vi "Sequencer.vi"(0 "Test (Default) en entrée":refnum<class "Sequencer (Default).lvclass">, 11 "error in (no error)":errorcluster caption="entrée d'erreur (pas d'erreur)") -> (4 "Test (Default) en sortie":refnum<class "Sequencer (Default).lvclass">, 6 "Json_String":string, 8 "Result":bool, 10 "Result Sequence":T3(array[cluster]), 15 "error out":errorcluster caption="sortie d'erreur")   [LabVIEW 2020, in "Library Core.lvlib" / "Sequencer (Default).lvclass"]
uses:
  Sequencer (Default).lvclass
  Commun VI/TypeDef/Commande Test/Commande Value Type.ctl
  Commun VI/TypeDef/Commande Test/Commande Type Test.ctl
  Actor Test (Default)/Actor Test (Default).lvclass
  Sequencer (Default).lvclass/Sequencer (Default).ctl
  Commun VI/TypeDef/Variable Printable.ctl
  Actor Test Firebase/Actor Test Firebase.lvclass
  C:/Users/ngarcin/OneDrive - Altyor/Standard TB/Suite TB45/Class/Sequencer/Actor Test (Default)/Actor Test (Default).lvclass
  Actor Test Database/Actor Test Database.lvclass
  Variable Test.vi
  Commun VI/Library Commun.lvlib
panel:
  out "Stop in progress":bool
  in  "Default":refnum<class "Actor Test (Default).lvclass">
  out "Numérique":i32
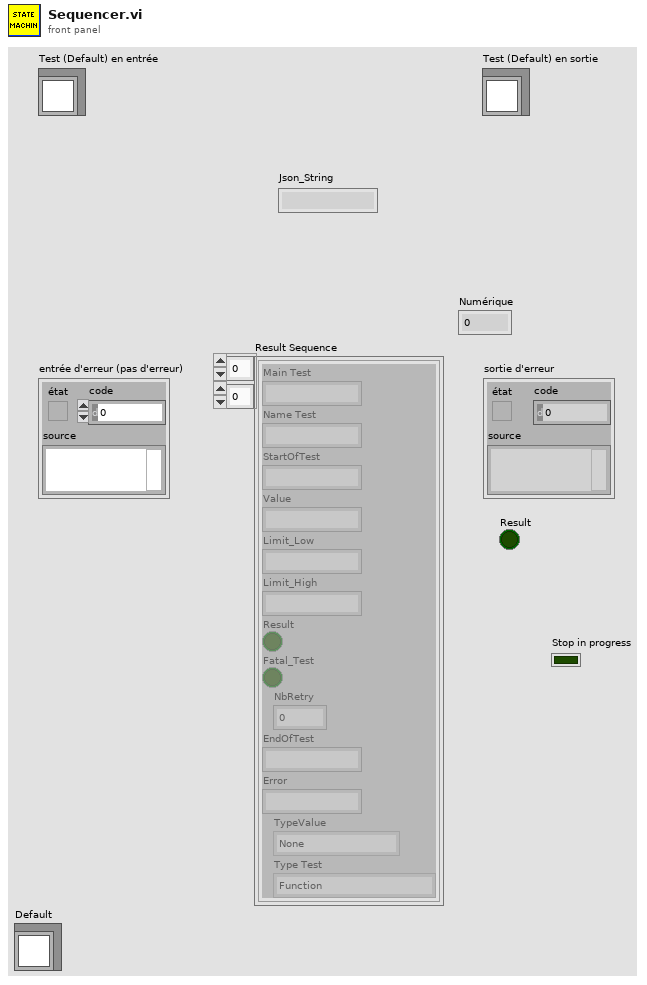
[diagram p1: front panel]
types:
  T1 = typedef "Library Commun.lvlib/Commande Value Type.ctl" = enum16{"None", "String", "Number", "Timestamp", "Boolean", "Array"}
  T2 = typedef "Library Commun.lvlib/Commande Type Test.ctl" = enum16{"Function", "Test", "Calculation"}
  T3 = cluster{"Main Test":string, "Name Test":string, "StartOfTest":string, "Value":string, "Limit_Low":string, "Limit_High":string, "Result":bool, "Fatal_Test":bool, "NbRetry":dbl, "EndOfTest":string, "Error":string, "TypeValue":T1, "Type Test":T2}[][]
  T4 = typedef "Variable Printable.ctl" = string
  T5 = enum16{"Get Variable", "Get All Variables", "Set Variable", "Delete Variable", "Delete All Variable"}
  T6 = enum16{"Get Actor Class", "Set Actor object", "Get Actor object", "List Actor", "Init"}
  T7 = typedef "Library Commun.lvlib/Actor Type.ctl" = enum16{"Default", "Firebase", "Database"}
  T8 = cluster{"Group Name":string, "Tab Test":cluster{"Type Function":string, "Test Name":string, "Class launched by the actors ":string, "Name_Instrument":string, "Class_Instrument":string, "Parameter (Json)":string, "Limit_Low":string, "Limit_Hight":string, "Fatal Test ?":bool, "Parallelized ?":bool, "Mandatory ?":bool}[], "Parallelized ?":bool, "Mandatory ?":bool}[]
  T9 = cluster{"Event Error":refnum<user-event>, "Data test ":refnum<user-event>, "Stop":refnum<user-event>, "Action in progress":refnum<user-event>, "Operator Shutdown":refnum<user-event>}
  T10 = cluster{"Type Function":string, "Test Name":string, "Class launched by the actors ":string, "Name_Instrument":string, "Class_Instrument":string, "Parameter (Json)":string, "Limit_Low":string, "Limit_Hight":string, "Fatal Test ?":bool, "Parallelized ?":bool, "Mandatory ?":bool}[]
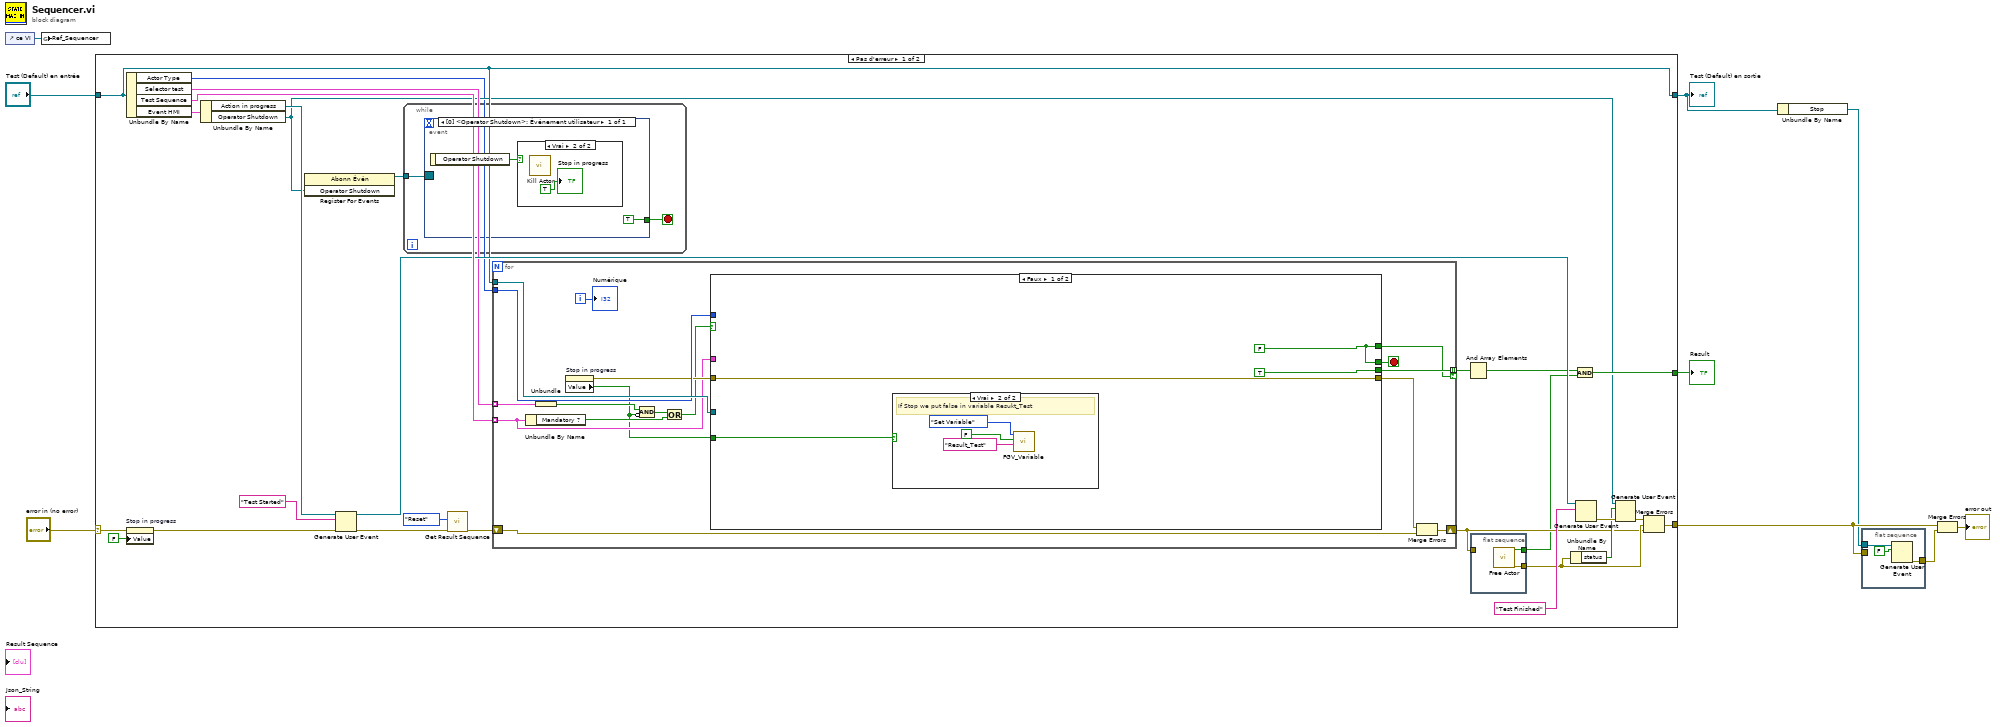
[diagram p0: block diagram]
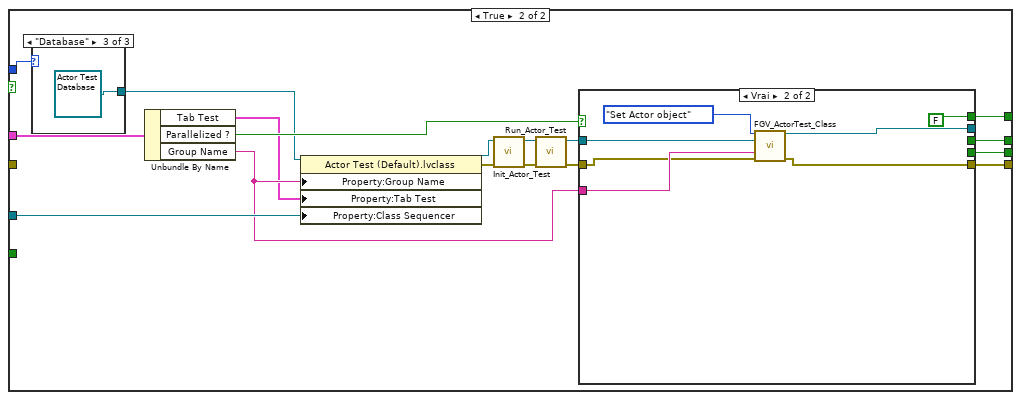
[diagram p3: hidden frame]
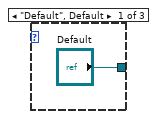
[diagram p4: hidden frame]
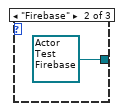
[diagram p5: hidden frame]
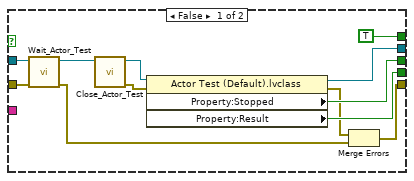
[diagram p6: hidden frame]
diagram:
  n1 = control-ref of="ce VI"() -> (w7:refnum<vi>)
  n2 = global write "Variable Test.vi" "Ref_Sequencer"(w7) -> ()
  n3 = case shown="Pas d'erreur" "error in (no error)" {
    selector: "error in (no error)" -> [w19 w108]
    tunnel: [w22 w108] -> w5
    tunnel: [w30 w107] -> w6
    tunnel: "Test (Default) en entrée" -> [w30 w107]
    tunnel: [w29 _] -> w2
    frame No Error {
      n4 = Unbundle By Name(w30) -> ("Actor Type"=w23:T7, "Selector test"=w28:cluster{"Booléen 4":bool}[], "Test Sequence"=w36:T8, "Event HMI"=w31:T9)
      n5 = property on="Stop in progress" class="Bool (strict)"(error in=w19, "Value"=FALSE ("Stop in progress")) -> (error out=w18:errorcluster)  [unwired: 1 in, 1 out]
      n6 = Unbundle By Name(w31) -> ("Action in progress"=w35:refnum<user-event>, "Operator Shutdown"=w24:refnum<user-event>)
      n7 = register-events(w24) -> (reference out=w27:refnum<event-registration>)  [unwired: 2 in, 1 out]
      n8 = Generate User Event(user event=w35, event data cluster="Test Started" ("données d'événement"), error in=w18) -> (user event out=w33:refnum<user-event>, error out=w15:errorcluster)  [unwired: 1 in]
      n9 = while {
        tunnel: w27 -> [w103]
        stop <- w102 stop-if-true
        n10 = event shown="[0] <Operator Shutdown>: Événement utilisateur" {
          selector: w103 -> [_]
          dyn-events: _ -> [_]
          timeout: _ -> [_]
          tunnel: [TRUE] -> w102
          event User Event {
            n11 = event-data() -> ("Operator Shutdown"=w105:bool)  [unwired: 1 in]
            n12 = case shown="Vrai" w105 {
              frame False {
              }
              frame True {
                n13 = call "Kill Actor.vi"() -> ()  [unwired: 11 in, 1 out]
                "Stop in progress" <- TRUE ("notification")
              }
            }
          }
        }
      }
      n14 = call "Get Result Sequence.vi"("error in (no error)"=w15, "Function"=enum16{"Get Result", "Reset", "Set Result"}."Reset") -> ("error out"=w14:errorcluster)  [unwired: 8 in, 1 out]
      n15 = for {
        shift-right: [w42] -> w13
        shift-left: w14 -> [w41]
        tunnel: w36 -> [w47] mode=indexing
        tunnel: w30 -> [w55]
        tunnel: w28 -> [w54] mode=indexing
        tunnel: [w52] -> w10 mode=indexing if=w51
        tunnel: w23 -> [w49]
        i -> [w50]
        stop <- w53 stop-if-true
        n16 = Unbundle By Name(w47) -> ("Mandatory ?"=w45:bool)
        n17 = Unbundle(w54) -> ("Booléen 4"=w40:bool)
        n18 = property on="Stop in progress" class="Bool (strict)"() -> (error out=w48:errorcluster, "Value"=w39:bool)  [unwired: 2 in, 1 out]
        n19 = Compound Arithmetic op=AND ("Opérateur arithmétique")(w40, invert w39) -> (w46:bool)
        n20 = Or(x=w46, y=w45) -> (x .or. y?=w44:bool)
        n21 = case shown="Faux" w44 {
          tunnel: w47 -> [_ w79]
          tunnel: w48 -> [w59 _]
          tunnel: w55 -> [_ w72]
          tunnel: [w59 w66] -> w43
          tunnel: [w57 w70] -> w53
          tunnel: [TRUE ("Property:Result") w71] -> w52
          tunnel: [w57 w69] -> w51
          tunnel: w49 -> [_ w64]
          tunnel: w39 -> [w56 _]
          frame False {
            w57 = FALSE ("Property:Stopped")
            n22 = case shown="Vrai" w56 {
              frame False {
              }
              frame True {
                # "If Stop we put false in variable Resukt_Test"
                n23 = call "FGV_Variable.vi"("Variable"=T4 "Result_Test", "Data In"=FALSE ("Affiche result"), "Function"=T5."Set Variable") -> ()  [unwired: 6 in, 3 out]
              }
            }
          }
          frame True {
            n24 = case shown="\"Database\"" w64 {
              tunnel: ["Default" refnum<class "Actor Test Firebase.lvclass"> refnum ("Library Sequencer.lvlib:Actor Test Firebase.lvclass") refnum<class "Actor Test Database.lvclass"> refnum ("Library Sequencer.lvlib:Actor Test Database.lvclass")] -> w67
              frame "Default", Default {
              }
              frame "Firebase" {
              }
              frame "Database" {
              }
            }
            n25 = Unbundle By Name(w79) -> ("Tab Test"=w63:T10, "Parallelized ?"=w68:bool, "Group Name"=w65:string)
            n26 = property class="Actor Test (Default).lvclass"(reference=w67, "Property:Group Name"=w65, "Property:Tab Test"=w63, "Property:Class Sequencer"=w72) -> (reference out=w73:refnum<class "Actor Test (Default).lvclass">, error out=w74:errorcluster)  [unwired: 1 in]
            n27 = call-dynamic "Init_Actor_Test.vi"("error in (no error)"=w74, "Test (Default) en entrée"=w73) -> ("error out"=w75:errorcluster, "Test (Default) en sortie"=w76:refnum<class "Actor Test (Default).lvclass">)  [unwired: 8 in]
            n28 = call-dynamic "Run_Actor_Test.vi"("error in (no error)"=w75, "Test (Default) en entrée"=w76) -> ("error out"=w77:errorcluster, "Test (Default) en sortie"=w78:refnum<class "Actor Test (Default).lvclass">)  [unwired: 8 in]
            n29 = case shown="Vrai" w68 {
              tunnel: w78 -> [w94 w99]
              tunnel: w77 -> [w93 w96]
              tunnel: [w86 w95] -> w66
              tunnel: [w91 w97] -> _
              tunnel: [w90 _] -> w71
              tunnel: [w89 _] -> w70
              tunnel: [TRUE FALSE] -> w69
              tunnel: w65 -> [_ w98]
              frame False {
                n30 = call-dynamic "Wait_Actor_Test.vi"("error in (no error)"=w93, "Test (Default) en entrée"=w94) -> ("error out"=w85:errorcluster, "Test (Default) en sortie"=w84:refnum<class "Actor Test (Default).lvclass">)  [unwired: 8 in]
                n31 = call-dynamic "Close_Actor_Test.vi"("Test (Default) en entrée"=w84) -> ("error out"=w83:errorcluster, "Test (Default) en sortie"=w92:refnum<class "Actor Test (Default).lvclass">)  [unwired: 9 in]
                n32 = property class="Actor Test (Default).lvclass"(reference=w92, error in=w83) -> (reference out=w91:refnum<class "Actor Test (Default).lvclass">, error out=w87:errorcluster, "Property:Stopped"=w89:bool, "Property:Result"=w90:bool)
                n33 = Merge Errors(w87, w85) -> (w86:errorcluster)
              }
              frame True {
                n34 = call "FGV_ActorTest_Class.vi"("Action"=T6."Set Actor object", "Actor Test"=w99, "Group Name"=w98, "error in (no error)"=w96) -> ("Actor Test"=w97:refnum<class "Actor Test (Default).lvclass">, "error out"=w95:errorcluster)  [unwired: 8 in, 2 out]
              }
            }
          }
        }
        n35 = Merge Errors(w43, w41) -> (w42:errorcluster)
        "Numérique" <- w50
      }
      n36 = And Array Elements(Boolean array=w10) -> (logical AND=w11:bool)
      n37 = flat-sequence {
        tunnel: [w38] -> w12
        tunnel: w13 -> [_]
        tunnel: [w37] -> w21
        frame #0 {
          n38 = call "Free Actor.vi"() -> ("error out"=w37:errorcluster, "Result"=w38:bool)  [unwired: 10 in]
        }
      }
      n39 = Unbundle By Name(w21) -> ("status"=w20:bool)
      n40 = And(x=w11, y=w12) -> (x .and. y?=w29:bool)
      n41 = Generate User Event(user event=w33, event data cluster="Test Finished" ("données d'événement")) -> (error out=w26:errorcluster)  [unwired: 2 in, 1 out]
      n42 = Generate User Event(user event=w24, event data cluster=w20, error in=w26) -> (error out=w25:errorcluster)  [unwired: 1 in, 1 out]
      n43 = Merge Errors(w25, w21, w13) -> (w22:errorcluster)
    }
    frame Error {
    }
  }
  "Test (Default) en sortie" <- w6
  "Result" <- w2
  n44 = Unbundle By Name(w6) -> ("Stop"=w1:refnum<user-event>)
  n45 = flat-sequence {
    tunnel: w5 -> [_]
    tunnel: [w111] -> w4
    tunnel: w1 -> [w110]
    frame #0 {
      n46 = Generate User Event(user event=w110, event data cluster=FALSE ("données d'événement")) -> (error out=w111:errorcluster)  [unwired: 2 in, 1 out]
    }
  }
  n47 = Merge Errors(w5, w4) -> (→"error out":errorcluster)
